vi "WSVCAP SHL Host TL RFFE Stop Write Cycle.vi"(11 "error in":errorcluster, 14 "Log (T)":bool=TRUE) -> (15 "error out":errorcluster)   [LabVIEW 2012]
uses:
  Type Defs/WSVCAP SHL Function Enum.ctl
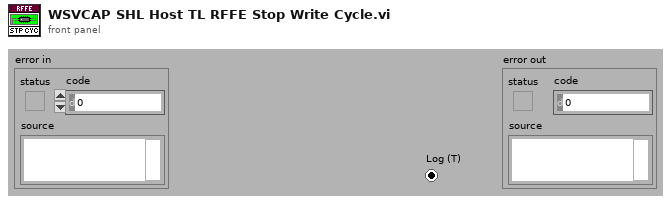
[diagram p1: front panel]
types:
  T1 = typedef "WSVCAP SHL Function Enum.ctl" = enum16{"Initialize", "Configure I2C", "Configure SPI", "Configure RFFE", "Write I2C", "Read I2C", "Write/Read SPI", "Start SPI Cycle", "Stop SPI Cycle", "Write RFFE", "Read RFFE", "Start RFFE Cycle", "Stop RFFE Cycle", "Get Status", "Close"}
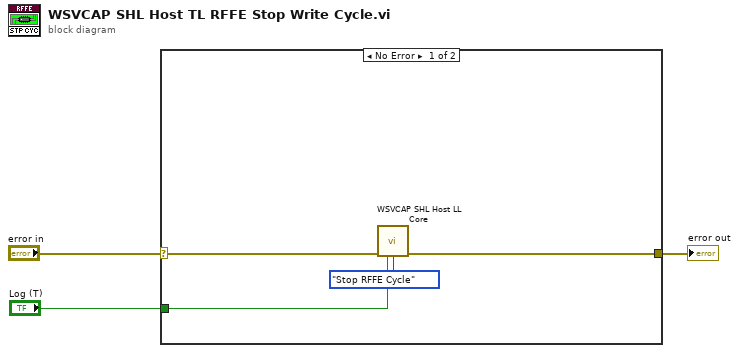
[diagram p0: block diagram]
diagram:
  n1 = case shown="No Error" "error in" {
    selector: "error in" -> [w6 _]
    tunnel: [w5 _] -> w3
    tunnel: "Log (T)" -> [w4 _]
    frame No Error {
      n2 = call "WSVCAP SHL Host LL Core.vi"("error in"=w6, "Log (T)"=w4, "Function"=WSVCAP_SHL_Function_Enum."Stop RFFE Cycle") -> ("error out"=w5:errorcluster)  [unwired: 10 in, 2 out]
    }
    frame Error {
    }
  }
  "error out" <- w3
